vi "shiftlevervoltagetest.vi"() -> ()   [LabVIEW 2015]
uses:
  <vilib>/myRIO/Common/Instrument Driver Framework/myRIO v1.0/DIO/vis/myRIO v1.0 Close DIO.vi
  <vilib>/myRIO/Common/Instrument Driver Framework/myRIO v1.0/AO/vis/myRIO v1.0 Close AO.vi
  <vilib>/myRIO/Common/Instrument Driver Framework/myRIO v1.0/DIO/vis/myRIO v1.0 Unreserve DIO.vi
  <vilib>/myRIO/Common/Instrument Driver Framework/myRIO v1.0/AO/vis/myRIO v1.0 Unreserve AO.vi
  <vilib>/myRIO/Common/Instrument Driver Framework/myRIO v1.0/DIO/vis/myRIO v1.0 Build MUX Configuration DIO.vi
  <vilib>/myRIO/Common/Instrument Driver Framework/myRIO v1.0/Resource Manager/vis/myRIO v1.0 Unreserve Channel List.vi
  <vilib>/myRIO/Common/Instrument Driver Framework/myRIO v1.0/AO/vis/myRIO v1.0 Build MUX Configuration AO.vi
  <vilib>/myRIO/Common/Instrument Driver Framework/myRIO v1.0/Resource Manager/vis/myRIO v1.0 Create Configuration List.vi
  <vilib>/myRIO/Common/Instrument Driver Framework/myRIO v1.0/Resource Manager/vis/myRIO v1.0 Unreserve Channel.vi
  <vilib>/myRIO/Common/Instrument Driver Framework/myRIO v1.0/Resource Manager/vis/myRIO v1.0 Build Mutex Name.vi
  <vilib>/Utility/error.llb/Error Cluster From Error Code.vi
  <vilib>/myRIO/Common/Instrument Driver Framework/myRIO v1.0/DIO/vis/myRIO v1.0 Write DIO.vi
  <vilib>/myRIO/Common/Instrument Driver Framework/myRIO v1.0/AO/vis/myRIO v1.0 Write AO.vi
  <vilib>/myRIO/Common/Instrument Driver Framework/myRIO v1.0/DIO/vis/myRIO v1.0 Shutdown DIO.vi
  <vilib>/myRIO/Common/Instrument Driver Framework/myRIO v1.0/Resource Manager/vis/myRIO v1.0 Configure IO.vi
  <vilib>/myRIO/Common/Instrument Driver Framework/Utilities/vis/Configuration Manager.vi
  <vilib>/myRIO/Common/Instrument Driver Framework/Utilities/vis/IO Manager.vi
  <vilib>/myRIO/Common/Instrument Driver Framework/myRIO v1.0/myRIO v1.0 Close.vi
  <vilib>/myRIO/Instrument Drivers/Onboard IO/AO/AO.lvlib
  <vilib>/myRIO/Instrument Drivers/Onboard IO/DIO/DIO.lvlib
panel:
  in  "Ring":u16(ring) items=["R", "N", "D"]
  in  "Shift":bool=TRUE
  out "error out":errorcluster
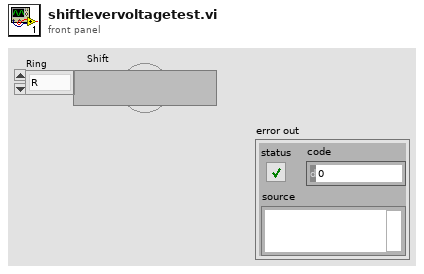
[diagram p1: front panel]
types:
  T1 = typedef "AO.lvlib/AO Reference.ctl" = cluster{"myRIO Reference":T2, "AO Channel List":T6, "AO Scaling Constant List":T8}
  T2 = typedef "myRIO Generic Hardware Reference.ctl" = cluster{"myRIO Model":T3, "myRIO Hardware Reference":T4}
  T3 = typedef "Hardware Version Enum.ctl" = enum16{"Unknown", "myRIO-1900", "myRIO-1950", "roboRIO"}
  T4 = typedef "myRIO v1.0 Reference.ctl" = cluster{"Generic FPGA Reference":T5, "Allow multiple opens":bool}
  T5 = typedef "Generic FPGA Reference.ctl" = refnum<k20>
  T6 = typedef "AO Channels List.ctl" = T7[]
  T7 = typedef "AO Channels Enum.ctl" = enum16{"Not Connected", "AudioOut/Left", "AudioOut/Right", "C/AO0", "C/AO1", "A/AO0", "A/AO1", "B/AO0", "B/AO1"}
  T8 = typedef "Analog Scaling Constants List.ctl" = T9[]
  T9 = typedef "Analog Scaling Constants.ctl" = cluster{"LSB Weight (Volts)":dbl, "Offset (Volts)":dbl, "Signed?":bool}
  T10 = typedef "DIO.lvlib/DIO Reference.ctl" = cluster{"myRIO Reference":T2, "DIO Channels List":T11}
  T11 = typedef "DIO Channels List.ctl" = T12[]
  T12 = typedef "DIO Channels Enum.ctl" = enum16{"Not Connected", "C/DIO0", "C/DIO1", "C/DIO2", "C/DIO3", "C/DIO4", "C/DIO5", "C/DIO6", "C/DIO7", "A/DIO0", "A/DIO1", "A/DIO2", "A/DIO3", "A/DIO4", "A/DIO5", "A/DIO6", "A/DIO7", "A/DIO8", "A/DIO9", "A/DIO10", "A/DIO11", "A/DIO12", "A/DIO13", "A/DIO14", "A/DIO15", "B/DIO0", "B/DIO1", "B/DIO2", "B/DIO3", "B/DIO4", "B/DIO5", "B/DIO6", "B/DIO7", "B/DIO8", "B/DIO9", "B/DIO10", "B/DIO11", "B/DIO12", "B/DIO13", "B/DIO14", "B/DIO15", "LED0", "LED1", "LED2", "LED3", "Button0", "DIO/DIO0", "DIO/DIO1", "DIO/DIO2", "DIO/DIO3", "DIO/DIO4", "DIO/DIO5", "DIO/DIO6", "DIO/DIO7", "DIO/DIO8", "DIO/DIO9", "SPI/CS0", "SPI/CS1", "SPI/CS2", "SPI/CS3", "LED RADIO (Green)", "LED RADIO (Red)", "LED COMM (Green)", "LED COMM (Red)", "LED MODE (Green)", "LED MODE (Red)"}
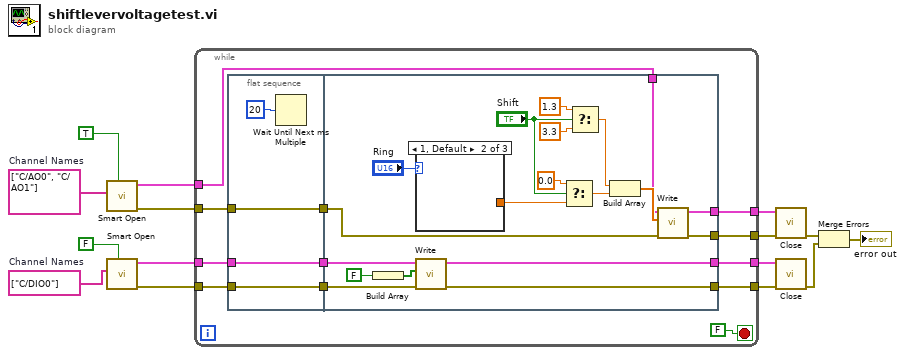
[diagram p0: block diagram]
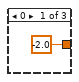
[diagram p2: hidden frame]
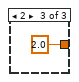
[diagram p3: hidden frame]
diagram:
  w10 = tag[] ["C/DIO0"]  # Channel Names
  w15 = tag[] ["C/AO0", "C/AO1"]  # Channel Names
  n1 = call <vilib>:"Smart Open.vi"("Allow multiple opens?"=TRUE, "Channel Names"=w15) -> ("error out"=w13:errorcluster, "AO Ref Out"=w14:T1)  [unwired: 8 in]
  n2 = call <vilib>:"Smart Open.vi"("Allow multiple opens?"=FALSE, "Channel Names"=w10) -> ("error out"=w6:errorcluster, "DIO Ref Out"=w9:T10)  [unwired: 8 in]
  n3 = while {
    tunnel: w14 -> [w27]
    tunnel: w13 -> [w26]
    tunnel: [w25] -> w12
    tunnel: [w23] -> w11
    tunnel: w9 -> [w18]
    tunnel: w6 -> [w20]
    tunnel: [w17] -> w5
    tunnel: [w16] -> w4
    stop <- FALSE stop-if-true
    n4 = flat-sequence {
      tunnel: w26 -> [w31]
      tunnel: [w31] -> w22
      tunnel: [w29] -> w21
      tunnel: w20 -> [w29]
      tunnel: [w28] -> w19
      tunnel: w18 -> [w28]
      tunnel: w27 -> [w49]
      tunnel: [w47] -> w25
      tunnel: [w46] -> w23
      tunnel: w22 -> [w48]
      tunnel: w21 -> [w37]
      tunnel: w19 -> [w36]
      tunnel: [w33] -> w17
      tunnel: [w32] -> w16
      frame #0 {
        n5 = Wait Until Next ms Multiple(millisecond multiple=u32 20) -> ()  [unwired: 1 out]
      }
      frame #1 {
        n6 = Build Array(FALSE ("NuLL (C/DIO0 (DIO0))")) -> (w34:bool[])
        n7 = case shown="1, Default" "Ring" {
          tunnel: [-2.0 _ 2.0] -> w40
          frame 0 {
          }
          frame 1, Default {
          }
          frame 2 {
          }
        }
        n8 = call <vilib>:"Write.vi"("error in (no error)"=w37, "Values"=w34, "DIO Ref In"=w36) -> ("error out"=w32:errorcluster, "DIO Ref Out"=w33:T10)  [unwired: 6 in]
        n9 = Select(t=0.0, s="Shift", f=w40) -> (s? t:f=w39:dbl)
        n10 = Select(t=1.3, s="Shift", f=3.3) -> (s? t:f=w43:dbl)
        n11 = Build Array(w43, w39) -> (w50:dbl[])
        n12 = call <vilib>:"Write.vi"("error in (no error)"=w48, "Values"=w50, "AO Ref In"=w49) -> ("error out"=w47:errorcluster, "AO Ref Out"=w46:T1)  [unwired: 6 in]
      }
    }
  }
  n13 = call <vilib>:"Close.vi"("error in (no error)"=w12, "AO Ref In"=w11) -> ("error out"=w3:errorcluster)  [unwired: 9 in]
  n14 = call <vilib>:"Close.vi"("error in (no error)"=w4, "DIO Ref In"=w5) -> ("error out"=w2:errorcluster)  [unwired: 9 in]
  n15 = Merge Errors(w3, w2) -> (→"error out":errorcluster)
